vi "filter.vi"(11 "Numeric":u16) -> (2 "prevx 2":u16, 3 "prevx":u16)   [LabVIEW 2016]
uses:
  #defines.ctl
  GLOBALS.vi
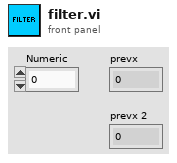
[diagram p1: front panel]
types:
  T1 = typedef "#defines.ctl" = i16
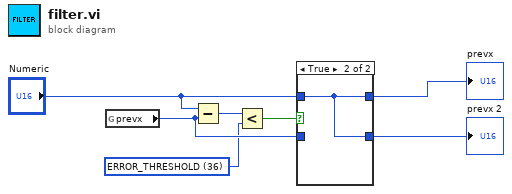
[diagram p0: block diagram]
diagram:
  w2 = T1 36 items=["ERROR_THRESHOLD"=36, "CTRL_REG9"=35, "STATUS_REG_1"=39, "OUT_X_L_XL"=40, "FIFO_CTRL"=46, "FIFO_SRC"=47, "CTRL_REG4"=30, "OUT_X_L_G"=24, "OUT_TEMP_L"=21, "INT_GEN_SRC_G"=20, "ORIENT_CFG_G"=19, "CTRL_REG3_G"=18, "CTRL_REG2_G"=17, "CTRL_REG1_G"=16, "WHO_AM_I_XG"=15] ("Ring")
  n1 = global read "GLOBALS.vi" "prevx"() -> (w7:i16)
  n2 = Subtract(x="Numeric", y=w7) -> (x-y=w1:u16)
  n3 = Less?(x=w1, y=w2) -> (x < y?=w3:bool)
  n4 = case shown="True" w3 {
    tunnel: w7 -> [w8 _]
    tunnel: [w8 w9] -> w4
    tunnel: [w8 w9] -> w5
    tunnel: "Numeric" -> [_ w9]
    frame False {
    }
    frame True {
    }
  }
  "prevx" <- w5
  "prevx 2" <- w4
